vi "SerialComplexInteractive.vi"(4 "error in (no error)":errorcluster) -> (0 "error out":errorcluster)   [LabVIEW 2010]
panel:
  in  "baud rate (9600)":u32=9600
  in  "VISA resource name":refnum<visa-resource-name>="COM1"
  in  "Repeat buffer":string
  in  "Repeat":bool
  in  "Clear history buffer":bool
  out "History":string
  in  "Send":bool
  in  "Clear rx buffer":bool
  in  "exit":bool
  in  "Command":string
  out "Reply Received":string
  # "Driving the controller doesn't require anything this complex, \nbut it is included in case you need to do what it does.\nThis VI works like Hyperterminal in that it continuously\nreads from the serial port into a buffer. It does that by\nusing an event loop. To see this event loop, you have to \nscroll down in the block diagram. This works well for\ninteractive sessions, especially when the reply is long.\nFor example, try this command: INFO X"
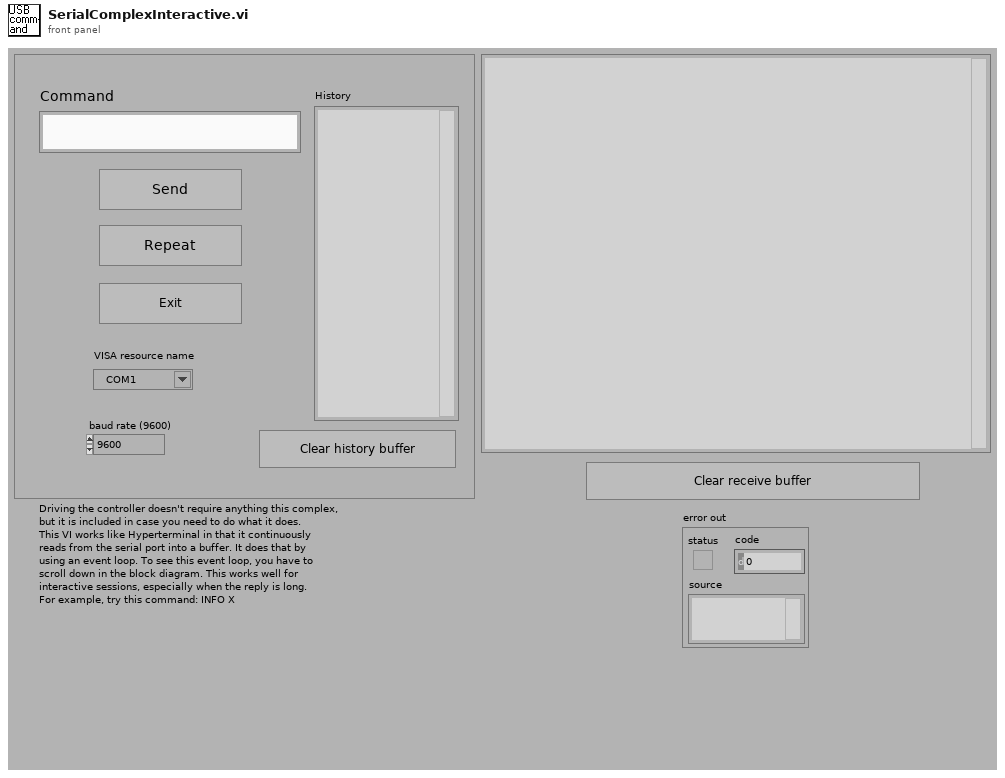
[diagram p1: front panel]
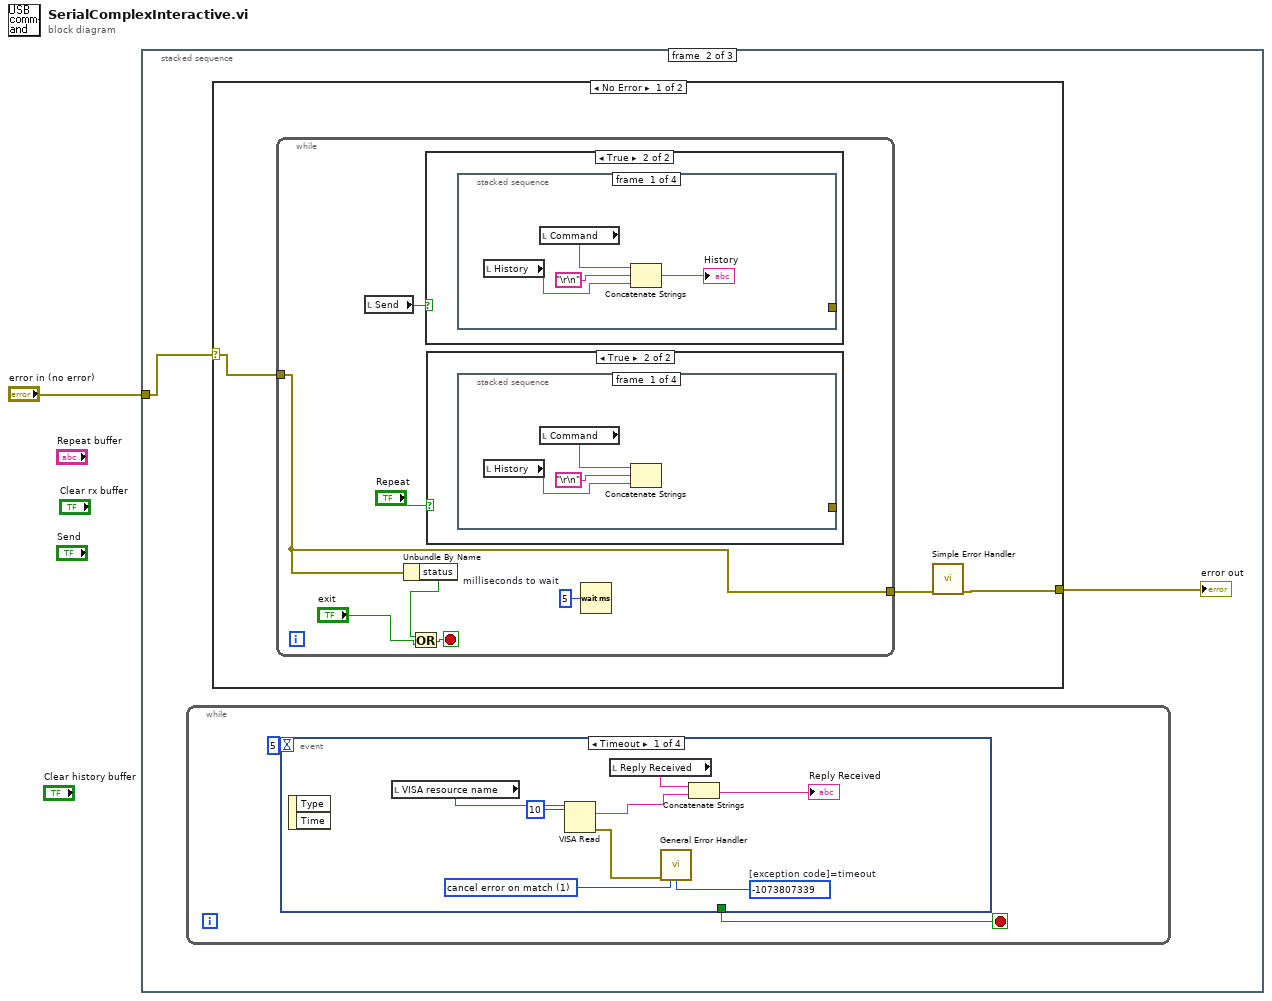
[diagram p0: block diagram]
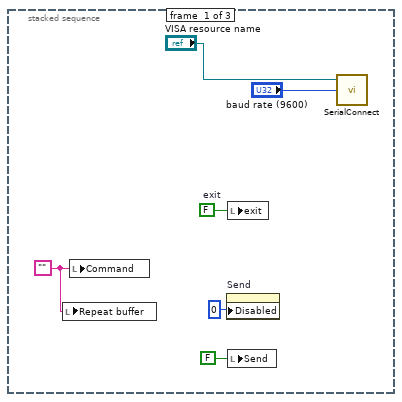
[diagram p2: hidden frame]
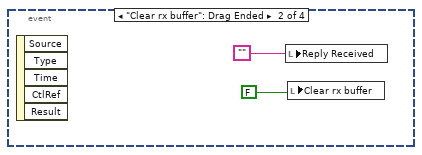
[diagram p3: hidden frame]
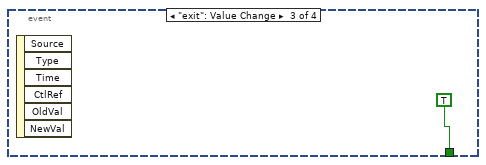
[diagram p4: hidden frame]
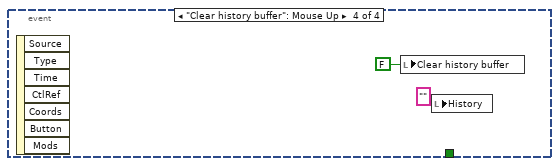
[diagram p5: hidden frame]
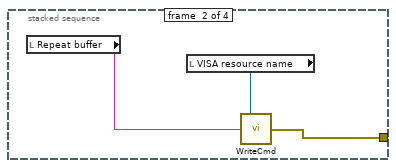
[diagram p7: hidden frame]
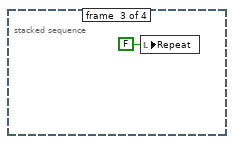
[diagram p8: hidden frame]
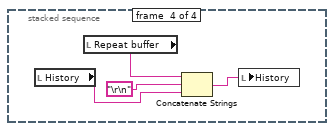
[diagram p9: hidden frame]
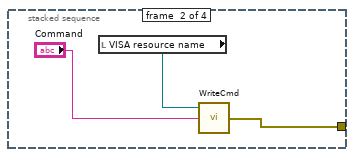
[diagram p11: hidden frame]
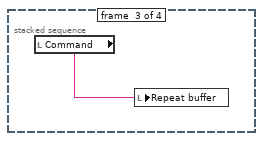
[diagram p12: hidden frame]
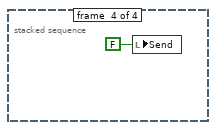
[diagram p13: hidden frame]
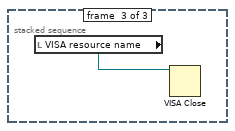
[diagram p15: hidden frame]
diagram:
  n1 = stacked-sequence {
    tunnel: "error in (no error)" -> [_ w8 _]
    frame #0 {
      w4 = ""
      w7 = FALSE  # exit
      n2 = local write "Repeat buffer"(w4) -> ()
      n3 = local write "Command"(w4) -> ()
      n4 = property on="Send" class="Bool (strict)"("Disabled"=u8 0) -> ()  [unwired: 2 in, 2 out]
      n5 = local write "exit"(w7) -> ()
      n6 = local write "Send"(FALSE ("Send")) -> ()
      n7 = call "SerialConnect.vi"("baud rate (9600)"="baud rate (9600)", "VISA resource name"="VISA resource name") -> ()  [unwired: 1 in, 3 out]
    }
    frame #1 {
      n8 = while {
        stop <- w11 stop-if-true
        n9 = event shown="[0] Timeout" {
          selector: _ -> [_ _ _ _]
          dyn-events: _ -> [_ _ _ _]
          timeout: 5 -> [_ _ _ _]
          tunnel: [_ _ TRUE _] -> w11
          event Timeout {
            w15 = 1 items=["no exception", "cancel error on match", "set error on match"] ("[exception action] (none:0)")
            w16 = -1073807339  # [exception code]=timeout
            n10 = event-data() -> ()  [unwired: 3 out]
            n11 = local read "VISA resource name"() -> (w19:refnum<visa-resource-name>)
            n12 = VISA Read(VISA resource name=w19, byte count=u32 10) -> (read buffer=w13:string, error out=w17:errorcluster)  [unwired: 1 in, 2 out]
            n13 = local read "Reply Received"() -> (w14:string)
            n14 = call <vilib>:"General Error Handler.vi"("error in (no error)"=w17, "[exception action] (none:0)"=w15, "[exception code]"=w16) -> ()  [unwired: 8 in, 5 out]
            n15 = Concatenate Strings "Concatenate Strings"(w14, w13) -> (→"Reply Received":string)
          }
          event "Clear rx buffer": Drag Ended {
            n16 = event-data() -> ()  [unwired: 6 out]
            n17 = local write "Reply Received"("") -> ()
            n18 = local write "Clear rx buffer"(FALSE) -> ()
          }
          event "exit": Value Change {
            n19 = event-data() -> ()  [unwired: 7 out]
          }
          event "Clear history buffer": Mouse Up {
            n20 = event-data() -> ()  [unwired: 8 out]
            n21 = local write "Clear history buffer"(FALSE ("Clear history buffer")) -> ()
            n22 = local write "History"("" ("History")) -> ()
          }
        }
      }
      n23 = case shown="No Error" w8 {
        selector: w8 -> [w27 w57]
        tunnel: [w25 w57] -> w9
        frame No Error {
          n24 = while {
            tunnel: w27 -> [w28]
            tunnel: [w28] -> w26
            stop <- w33 stop-if-true
            w34 = u32 5  # milliseconds to wait
            n25 = local read "Send"() -> (w30:bool)
            n26 = Unbundle By Name(w28) -> ("status"=w32:bool)
            n27 = Or(x=w32, y="exit") -> (x .or. y?=w33:bool)
            n28 = case shown="True" w30 {
              frame False {
              }
              frame True {
                n29 = stacked-sequence {
                  tunnel: [_ w53 _ _] -> _
                  frame #0 {
                    n30 = local read "History"() -> (w48:string)
                    n31 = local read "Command"() -> (w50:string)
                    n32 = Concatenate Strings "Concatenate Strings"(w50, "\r\n", w48) -> (→"History":string)
                  }
                  frame #1 {
                    n33 = local read "VISA resource name"() -> (w51:refnum<visa-resource-name>)
                    n34 = call "WriteCmd.vi"("Command"="Command", "VISA resource name"=w51) -> ("error"=w53:errorcluster)  [unwired: 1 in]
                  }
                  frame #2 {
                    n35 = local read "Command"() -> (w54:string)
                    n36 = local write "Repeat buffer"(w54) -> ()
                  }
                  frame #3 {
                    n37 = local write "Command"("" ("Command")) -> ()
                    n38 = local write "Send"(FALSE ("Send")) -> ()
                  }
                }
              }
            }
            n39 = case shown="True" "Repeat" {
              frame False {
              }
              frame True {
                n40 = stacked-sequence {
                  tunnel: [_ w40 _ _] -> _
                  frame #0 {
                    n41 = local read "History"() -> (w36:string)
                    n42 = local read "Command"() -> (w37:string)
                    n43 = Concatenate Strings "Concatenate Strings"(w37, "\r\n", w36) -> ()  [unwired: 1 out]
                  }
                  frame #1 {
                    n44 = local read "Repeat buffer"() -> (w39:string)
                    n45 = local read "VISA resource name"() -> (w38:refnum<visa-resource-name>)
                    n46 = call "WriteCmd.vi"("Command"=w39, "VISA resource name"=w38) -> ("error"=w40:errorcluster)  [unwired: 1 in]
                  }
                  frame #2 {
                    n47 = local write "Command"("" ("Command")) -> ()
                    n48 = local write "Repeat"(FALSE ("Send")) -> ()
                  }
                  frame #3 {
                    n49 = local read "History"() -> (w45:string)
                    n50 = local read "Repeat buffer"() -> (w46:string)
                    n51 = Concatenate Strings(w46, "\r\n", w45) -> (w43:string)
                    n52 = local write "History"(w43) -> ()
                  }
                }
              }
            }
            n53 = Wait (ms)(milliseconds to wait=w34) -> ()  [unwired: 1 out]
          }
          n54 = call <vilib>:"Simple Error Handler.vi"("error in (no error)"=w26) -> ("error out"=w25:errorcluster)  [unwired: 1 in, 7 out]
        }
        frame Error {
        }
      }
      "error out" <- w9
    }
    frame #2 {
      n55 = local read "VISA resource name"() -> (w58:refnum<visa-resource-name>)
      n56 = VISA Close(VISA resource name=w58) -> ()  [unwired: 1 in, 1 out]
    }
  }
